vi "Get All Exchanges.vi"(8 "error in (no error)":errorcluster caption="entrée d'erreur (pas d'erreur)", 11 "Exchanges en entrée":refnum<class "Exchanges.lvclass"> caption="DNL_LabVIEW Object in") -> (0 "error out":errorcluster caption="sortie d'erreur", 1 "Exchanges":T1[](array[typedef]), 2 "Keys":variant[](array[variant]), 3 "Exchanges en sortie":refnum<class "Exchanges.lvclass"> caption="DNL_LabVIEW Object out", 4 "tableau a afficher":string[][](array[string]))   [LabVIEW 2012, in "Exchanges.lvclass"]
uses:
  Exchanges.lvclass
  Exchange/Exchange Parameters.ctl
  Exchange/Exchange Type Enum.ctl
  controls/Currencies.ctl
  Exchanges.lvclass/Exchanges.ctl
  Exchange/Exchange.lvclass
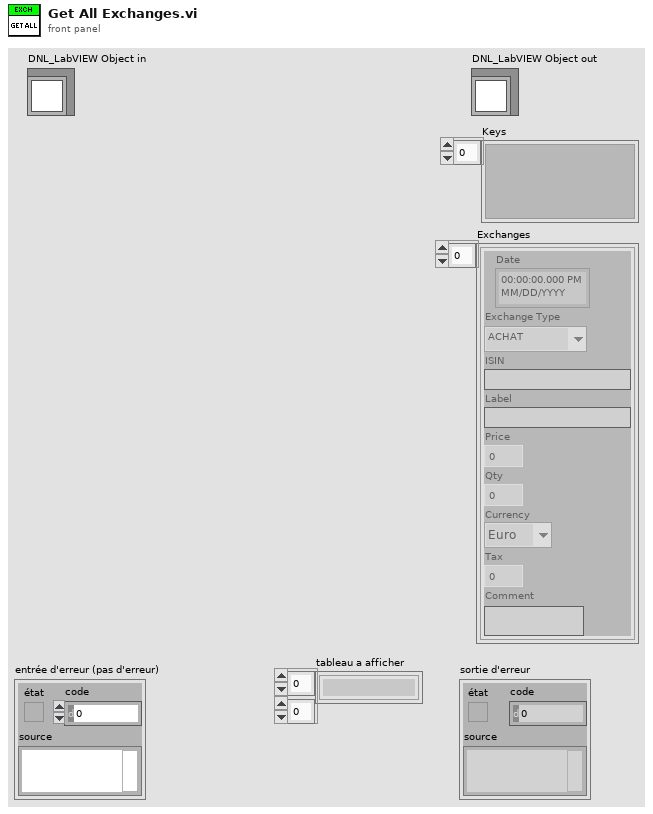
[diagram p1: front panel]
types:
  T1 = typedef "Exchange Parameters.ctl" = cluster{"Date":timestamp, "Exchange Type":T2, "ISIN":string, "Label":string, "Price":dbl, "Qty":dbl, "Currency":T3, "Tax":dbl, "Comment":string}
  T2 = typedef "Exchange.lvclass/Exchange Type Enum.ctl" = enum16{"ACHAT", "VENTE"}
  T3 = typedef "Currencies.ctl" = enum16{"Euro", "Dollar", "Yen", "RIM", "CHF"}
  T4 = typedef "Dictionary Object RefNum__ogtk.ctl" = refnum<k1>
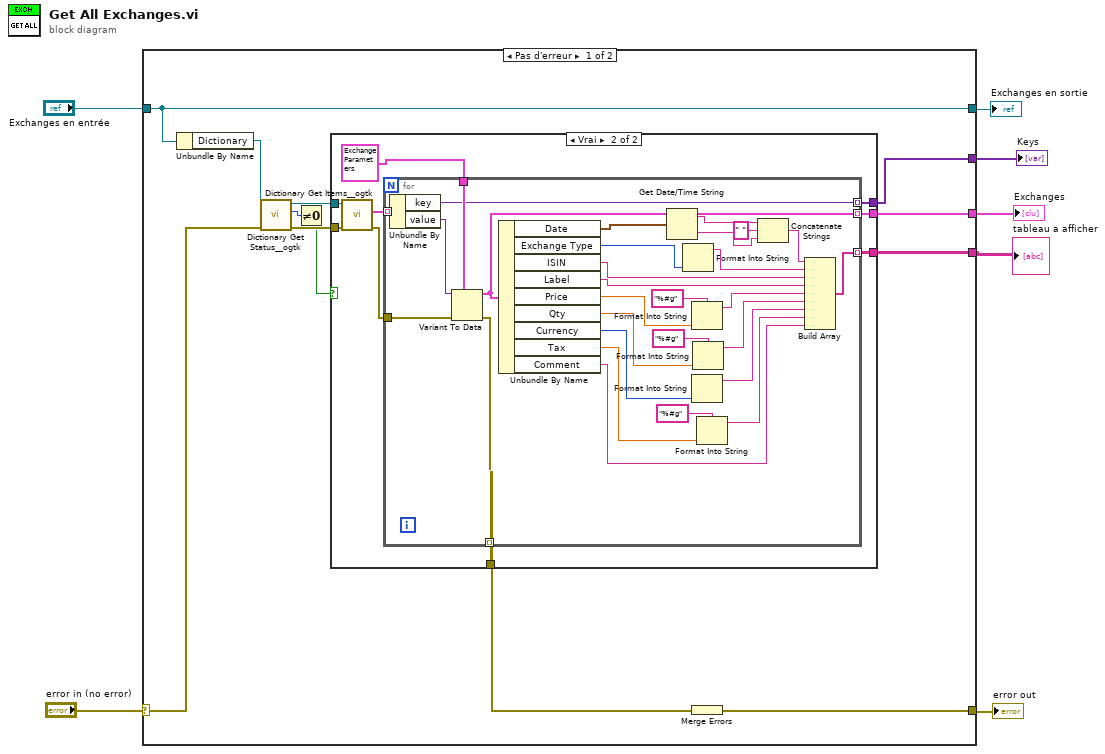
[diagram p0: block diagram]
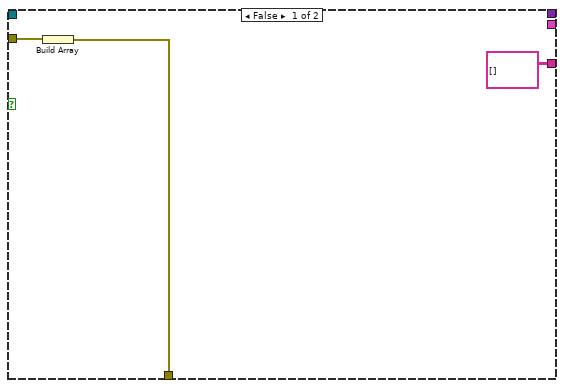
[diagram p2: hidden frame]
diagram:
  n1 = case shown="Pas d'erreur" "error in (no error)" {
    selector: "error in (no error)" -> [w13 w62]
    tunnel: [w10 w62] -> w6
    tunnel: [w14 w61] -> w4
    tunnel: "Exchanges en entrée" -> [w14 w61]
    tunnel: [w12 _] -> w3
    tunnel: [w9 _] -> w1
    tunnel: [w8 _] -> w2
    frame No Error {
      n2 = Unbundle By Name(w14) -> ("Dictionary"=w19:T4)
      n3 = call <userlib>:"Dictionary Get Status__ogtk.vi"("error in (no error)"=w13, "dictionary"=w19) -> ("error out"=w17:errorcluster, "size"=w16:i32, "dictionary out"=w18:T4)  [unwired: 7 in]
      n4 = Not Equal To 0?(x=w16) -> (x != 0?=w15:bool)
      n5 = case shown="Vrai" w15 {
        tunnel: w18 -> [_ w31]
        tunnel: w17 -> [w21 w30]
        tunnel: [w20 w27] -> w11
        tunnel: [_ w26] -> w9
        tunnel: [_ w25] -> w8
        tunnel: [string[][] [] w24] -> w12
        frame False {
          n6 = Build Array(w21) -> (w20:errorcluster[])
        }
        frame True {
          n7 = call <userlib>:"Dictionary Get Items__ogtk.vi"("error in (no error)"=w30, "dictionary"=w31) -> ("error out"=w28:errorcluster, "items"=w29:cluster{"key":variant, "value":variant}[])  [unwired: 7 in, 1 out]
          n8 = for {
            tunnel: w29 -> [w60] mode=indexing
            tunnel: T1 {"Date"=timestamp(0 s since 1904-01-01), "Exchange Type"=enum."ACHAT", "ISIN"="", "Label"="", "Price"=0.0, "Qty"=0.0, "Currency"=enum."Euro", "Tax"=0.0, "Comment"=""} ("Parameters") -> [w59]
            tunnel: w28 -> [w57]
            tunnel: [w56] -> w27 mode=indexing
            tunnel: [w54] -> w26 mode=indexing
            tunnel: [w55] -> w25 mode=indexing
            tunnel: [w50] -> w24 mode=indexing
            n9 = Unbundle By Name(w60) -> ("key"=w55:variant, "value"=w58:variant)
            n10 = Variant To Data(error in=w57, type=w59, Variant=w58) -> (data=w54:T1, error out=w56:errorcluster)
            n11 = Unbundle By Name(w54) -> ("Date"=w53:timestamp, "Exchange Type"=w51:T2, "ISIN"=w44:string, "Label"=w43:string, "Price"=w42:dbl, "Qty"=w39:dbl, "Currency"=w37:T3, "Tax"=w35:dbl, "Comment"=w32:string)
            n12 = Get Date/Time String(seconds (now)=w53) -> (date string=w52:string, time string=w47:string)  [unwired: 2 in]
            n13 = Format Into String(w51) -> (resulting string=w45:string)  [unwired: 3 in, 1 out]
            n14 = Format Into String(format string="%#g" ("chaîne de format"), w42) -> (resulting string=w41:string)  [unwired: 2 in, 1 out]
            n15 = Format Into String(w37) -> (resulting string=w34:string)  [unwired: 3 in, 1 out]
            n16 = Format Into String(format string="%#g" ("chaîne de format"), w39) -> (resulting string=w38:string)  [unwired: 2 in, 1 out]
            n17 = Format Into String(format string="%#g" ("chaîne de format"), w35) -> (resulting string=w33:string)  [unwired: 2 in, 1 out]
            n18 = Concatenate Strings(w52, " " ("chaîne"), w47) -> (w46:string)
            n19 = Build Array(w46, w45, w44, w43, w41, w38, w34, w33, w32) -> (w50:string[])
          }
        }
      }
      n20 = Merge Errors(w11) -> (w10:errorcluster)
    }
    frame Error {
    }
  }
  "error out" <- w6
  "Exchanges en sortie" <- w4
  "Exchanges" <- w1
  "Keys" <- w2
  "tableau a afficher" <- w3
